vi "Uframe-QImg-MNR.vi"() -> ()   [LabVIEW 2010]
uses:
  <vilib>/Platform/TimedLoop/XDataNode/XDataNode.xnode
  <vilib>/Platform/TimedLoop/XDataNode/timing_clust.ctl
  <vilib>/Platform/TimedLoop/XDataNode/nitl_modes.ctl
  <vilib>/Platform/TimedLoop/XDataNode/wakeup.ctl
  <vilib>/Platform/TimedLoop/XDataNode/XDNodeRunTimeDep.lvlib
panel:
  out "Current Exposure":dbl
  out "Current Offset":dbl(slide)=1080.0 min=0.0 max=4095.0 step=1.0 scale=0.0..4095.0
  out "Current Gain":dbl(slide)=1100.0 min=0.0 max=4095.0 step=1.0 scale=0.0..4095.0
  in  "AE":bool
  in  "Offset":dbl(slide)=1080.0 min=0.0 max=4095.0 step=1.0 scale=0.0..4095.0
  out "All Stop":bool=TRUE
  out "QImage":T1(plugin-control)
  in  "Gain":dbl(slide)=1100.0 min=0.0 max=4095.0 step=1.0 scale=0.0..4095.0
  in  "Exposure (ms)":dbl(slide)=100.0 min=1.6 max=10000.0 step=0.001 scale=1.6..10000.0
  out "Load Cell Constant (N/V)":dbl=44.48
  in  "Load Cell":u16(ring)=1 items=["440 N", "1250 N"]
  in  "Pause @ Load":bool
  in  "Pause @ N":dbl
  out "Disp (mm)":dbl
  out "Load (N)":dbl
  out "Image #":i32
  in  "Illumination":u32(ring) items=["White Light", "Flourescent"]
  in  "Timed \nAcquisition":bool
  out "Data Point":i32
  in  "Data \nAcquisition \nInterval (s)":dbl=1.0 min=0.1 max=60.0
  in  "Capture\nCurrent Image":bool
  in  "Max Load (N)":dbl=600.0 min=0.0 max=1200.0
  out "At Limit":bool
  in  "Rate Multiplier":dbl=1.0
  in  "Pause \nDisplacement":bool
  in  "Stop":bool
  in  "Invert \nDisplacement":bool
  in  "Zero \nDisplacement":bool=TRUE
  in  "Begin":bool
  out "Load vs Disp":cluster{dbl[], dbl[]}(graph)={[-724.1250113144533, -724.195323815552, -724.2656363166506, -724.3359488177492, -724.4062613188479, -724.4765738199465, -724.5468863210451, -724.6171988221438, -724.7461050741579, -724.9218863269045, -725.0976675796511, -725.2851675825808, -725.4492300851442], [-11.89350874713131, -11.896152101474941, -11.894229661847117, -11.89350874707076, -11.890865392620372, -11.895671491596438, -11.895911796524977, -11.899756675680168, -11.899035760801853, -11.90552399441818, -11.907927043887174, -11.905283689458143, -11.914655582386047]}
  out "Disp Vs Time":cluster{dbl[], dbl[]}(graph)={[-724.1250113144533, -724.195323815552, -724.2656363166506, -724.3359488177492, -724.4062613188479, -724.4765738199465, -724.5468863210451, -724.6171988221438, -724.7461050741579, -724.9218863269045, -725.0976675796511, -725.2851675825808, -725.4492300851442], [-11.89350874713131, -11.896152101474941, -11.894229661847117, -11.89350874707076, -11.890865392620372, -11.895671491596438, -11.895911796524977, -11.899756675680168, -11.899035760801853, -11.90552399441818, -11.907927043887174, -11.905283689458143, -11.914655582386047]}
  in  "File Name":string="Test"
  in  "File Path":path=path "C:/cygwin/home/Smarter Materials/Users 2015/Michael Rossol"
  in  "Sample Notes":string
  in  "Displacement \nRate (um/s)":dbl=3.0 min=3.0 max=50.0
  in  "Data Acquisition \nInterval (s)":dbl=1.0 min=0.1 max=10.0 step=0.01 format="%#_3g"
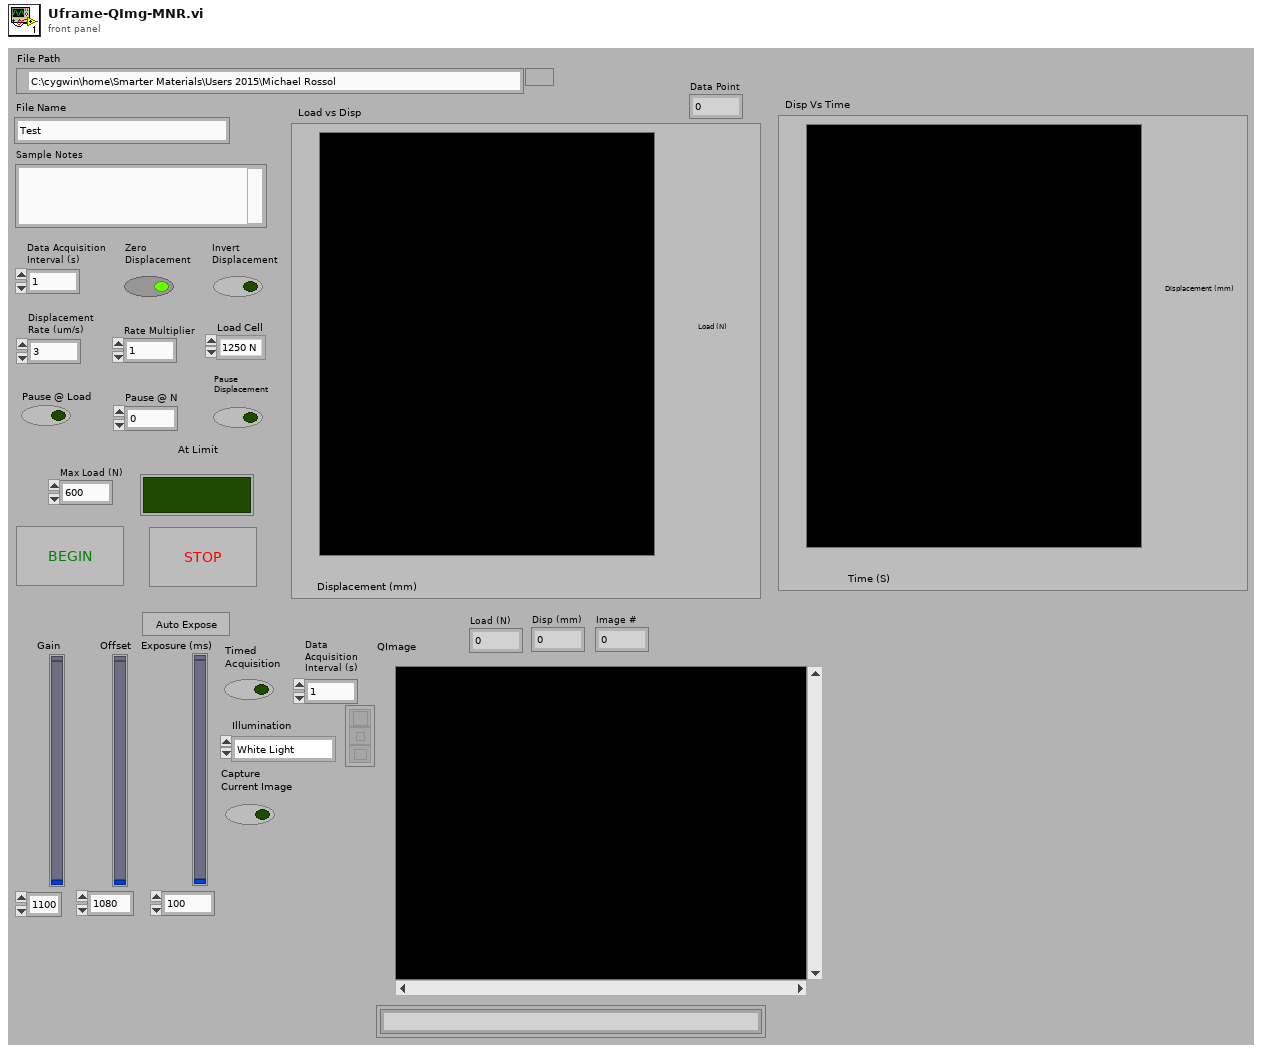
[diagram p1: front panel]
types:
  T1 = typedef "IMAQ Image.ctl" = refnum<image>
  T2 = enum32{"gain", "offset", "exposure", "binning", "horizontal binning", "vertical binning", "readout speed", "trigger type", "lcd filter", "cooler", "exposure red", "exposure blue", "image format", "roi x", "roi y", "roi width", "roi height", "reserved1", "shutter state", "reserved2", "sync-b out", "reserved3", "intensifier gain", "trigger delay", "camera mode", "normalized gain", "normalized intenifier gain DB", "doPostProcessing", "postProcessGainRed", "postProcessGainGreen", "postProcessGainBlue", "postProcessBayerAlgorithm", "postProcessImageFormat", "fan", "blackout mode", "high sensitivity", "Readout Port", "EM Gain", "open delay", "close delay", "clearing mode"}
  T3 = typedef "Image Type" = u32
  T4 = typedef "XDNodeRunTimeDep.lvlib/timing_clust.ctl" = cluster{"Expected End [f-1]":u64, "Actual End [f-1]":u64, "Finished Late? [f-1]":bool, "Expected End [i-1]":u64, "Actual End [i-1]":u64, "Finished Late? [i-1]":bool, "Expected Start [i]":u64, "Actual Start [i]":u64, "Expected Start [f]":u64, "Actual Start [f]":u64, "Source Name":string, "Structure Name":string, "Period":i64, "Deadline":i64, "Offset":i64, "Start":i64, "Priority":i32, "Timeout":i32, "Mode":T5, "Wakeup Reason":T6, "Error":errorcluster, "Source Type":string, "Secondary Source Type":string, "Global End Time":u64, "Global Start Time":u64, "Frame Duration":u64, "Iteration Duration":u64, "Assigned CPU":i32, "I/O Scan Engine Mode":u32}
  T5 = typedef "XDNodeRunTimeDep.lvlib/nitl_modes.ctl" = enum32{"No Change", "Process missed periods, maintain original phase", "Discard missed periods, maintain original phase", "Process missed periods, ignore original phase", "Discard missed periods, ignore original phase"}
  T6 = typedef "XDNodeRunTimeDep.lvlib/wakeup.ctl" = enum32{"Normal", "Aborted", "Asynchronous wakeup", "Timing source error", "Timed loop error", "Timeout"}
  T7 = cluster{"Global Rectangle":i32[], "Contours":cluster{"Contour Type":u32, "ROI Type":u32, "Points":i32[]}[]}
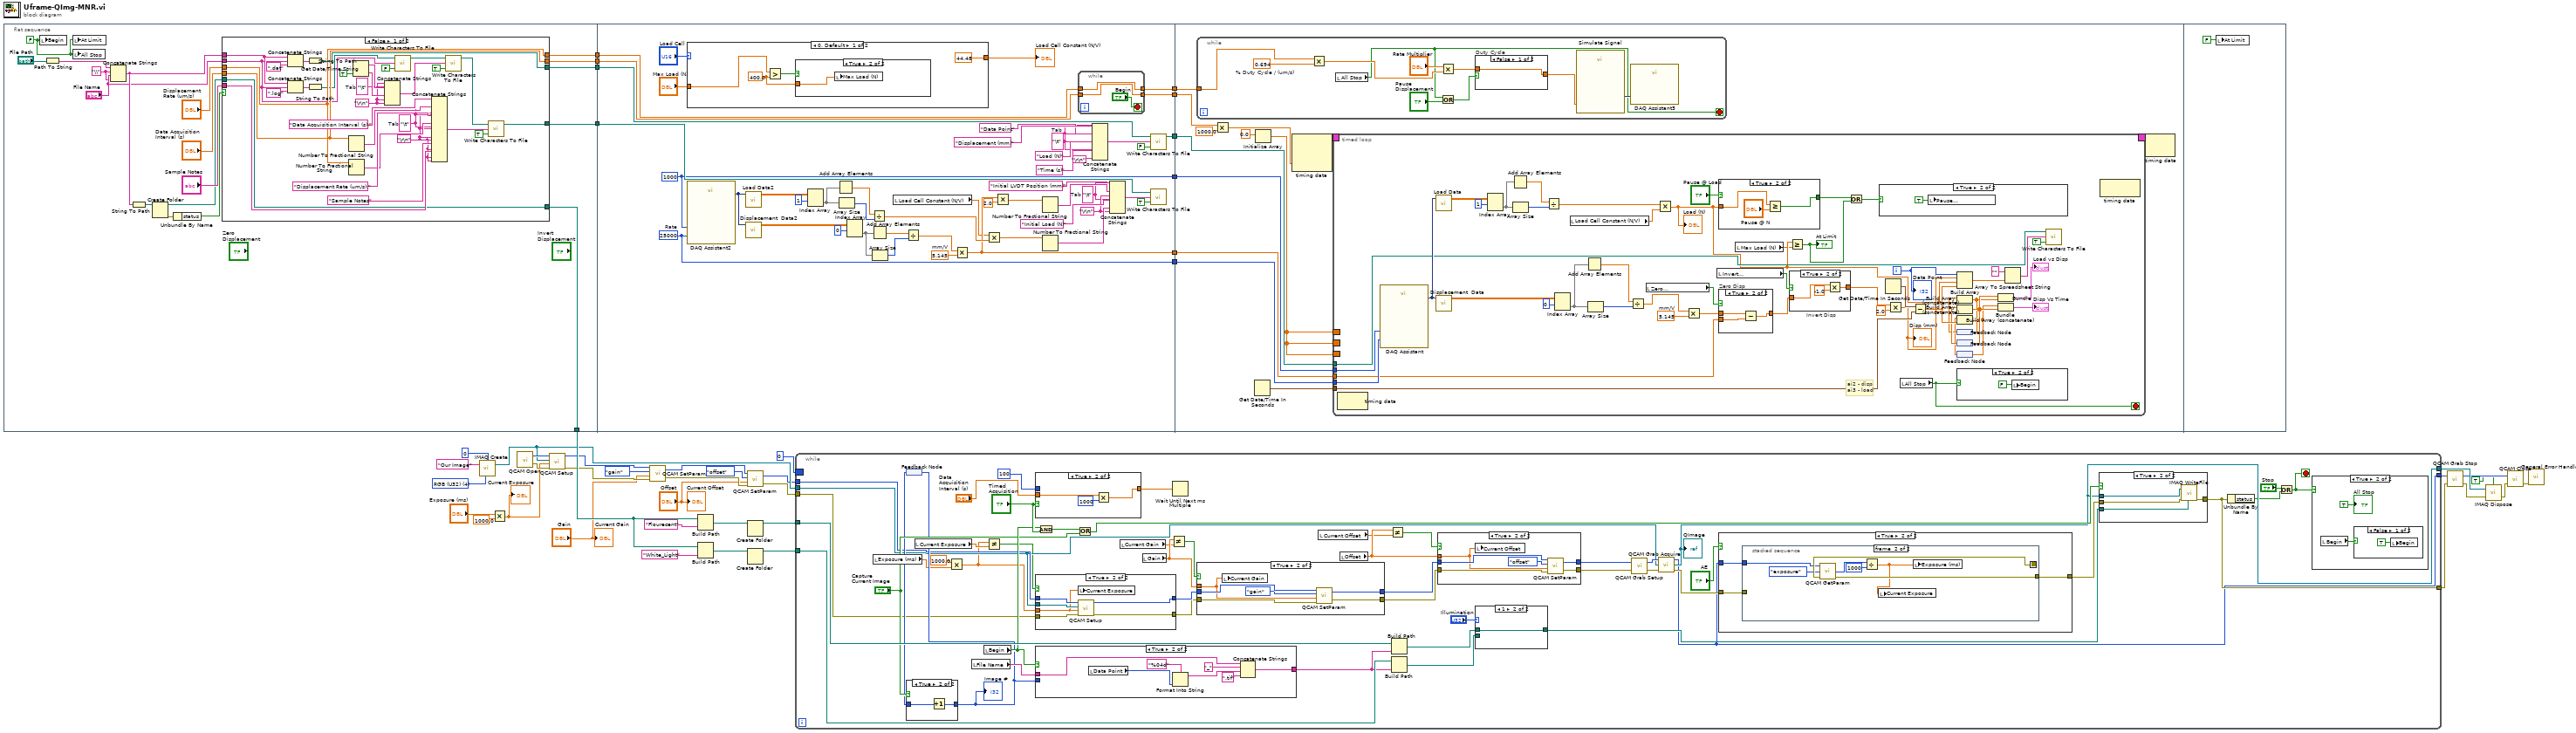
[diagram p0: block diagram]
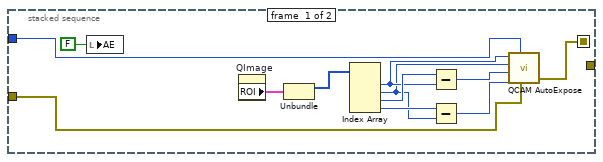
[diagram p6: hidden frame]
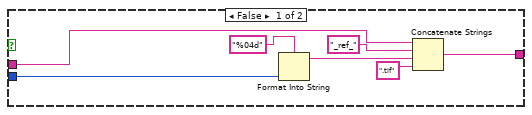
[diagram p10: hidden frame]
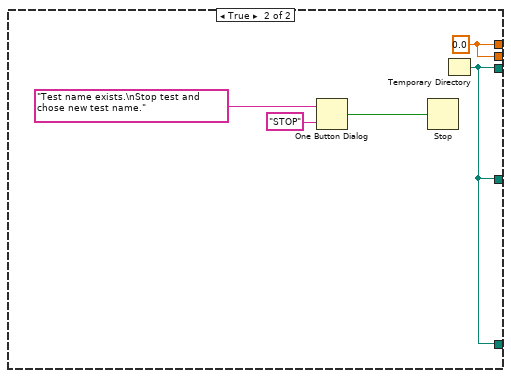
[diagram p14: hidden frame]
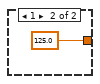
[diagram p16: hidden frame]
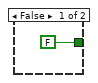
[diagram p17: hidden frame]
diagram:
  w21 = T3 4 items=["Grayscale (U8)", "Grayscale (I16)", "Grayscale (SGL)", "Complex (CSG)", "RGB (U32)", "HSL (U32)", "RGB (U64)"] ("Image Type")
  n1 = flat-sequence {
    tunnel: [w50] -> w41
    tunnel: [w62] -> w39
    tunnel: [w51] -> w38
    tunnel: [w52] -> w36
    tunnel: [w48] -> w29
    tunnel: [w105] -> w45
    tunnel: [w106] -> w44
    tunnel: [w107] -> w43
    tunnel: [w112] -> w42
    tunnel: w41 -> [w126]
    tunnel: [w117] -> w40
    tunnel: w39 -> [w116]
    tunnel: w38 -> [w109]
    tunnel: [w108] -> w37
    tunnel: w36 -> [w110]
    tunnel: w45 -> [w158]
    tunnel: w44 -> [w169]
    tunnel: w43 -> [w168]
    tunnel: w42 -> [w167]
    tunnel: w40 -> [w166]
    tunnel: w37 -> [w165]
    frame #0 {
      w49 = FALSE ("Begin")
      w47 = "\\"
      n2 = local write "Begin"(w49) -> ()
      n3 = Path To String(path="File Path") -> (string=w57:string)
      n4 = local write "At Limit"(w49) -> ()
      n5 = local write "All Stop"(w49) -> ()
      n6 = Concatenate Strings(w57, w47, "File Name", w47) -> (w55:string)
      n7 = String To Path(string=w55) -> (path=w59:path)
      n8 = Create Folder(path (use dialog)=w59) -> (created path=w46:path, error out=w58:errorcluster)  [unwired: 2 in, 1 out]
      n9 = Unbundle By Name(w58) -> ("status"=w56:bool)
      n10 = case shown="False" w56 {
        tunnel: [w81 w97] -> w50
        tunnel: "Data Acquisition \nInterval (s)" -> [w76 _]
        tunnel: "Displacement \nRate (um/s)" -> [w77 _]
        tunnel: "Sample Notes" -> [w73 _]
        tunnel: [w78 w97] -> w62
        tunnel: [w77 w96] -> w51
        tunnel: [w76 w96] -> w52
        tunnel: w55 -> [w66 _]
        tunnel: "File Name" -> [w65 _]
        tunnel: [w64 w97] -> w48
        tunnel: w46 -> [w64 _]
        frame False {
          w75 = "\t"  # Tab
          w72 = "\r\n"
          w91 = "\t"  # Tab
          w86 = "\r\n"
          n11 = Concatenate Strings(w66, w65, ".dat") -> (w79:string)
          n12 = Concatenate Strings(w66, w65, ".log") -> (w68:string)
          n13 = String To Path(string=w79) -> (path=w78:path)
          n14 = String To Path(string=w68) -> (path=w67:path)
          n15 = Number To Fractional String(number=w76) -> (F-format string=w84:string)  [unwired: 3 in]
          n16 = Number To Fractional String(number=w77) -> (F-format string=w82:string)  [unwired: 3 in]
          n17 = Get Date/Time String(want seconds? (F)=TRUE) -> (date string=w94:string, time string=w93:string)  [unwired: 2 in]
          n18 = Concatenate Strings(w86, w94, w91, w93, w86, w86) -> (w95:string)
          n19 = call <vilib>:"Write Characters To File.vi"("append to file? (new file:F)"=FALSE, "character string"=w65, "file path (dialog if empty)"=w67) -> ("new file path (Not A Path if cancelled)"=w71:path)  [unwired: 2 in]
          n20 = Concatenate Strings("Data Acquisition Interval (s):", w75, w84, w72, "Displacement Rate (um/s):", w75, w82, w72, w75, w72, w72, "Sample Notes", w72, w73, w72, w72) -> (w87:string)
          n21 = call <vilib>:"Write Characters To File.vi"("append to file? (new file:F)"=TRUE, "character string"=w95, "file path (dialog if empty)"=w71) -> ("new file path (Not A Path if cancelled)"=w89:path)  [unwired: 2 in]
          n22 = call <vilib>:"Write Characters To File.vi"("append to file? (new file:F)"=TRUE, "character string"=w87, "file path (dialog if empty)"=w89) -> ("new file path (Not A Path if cancelled)"=w81:path)  [unwired: 2 in]
        }
        frame True {
          w96 = 0.0 ("Displacement Rate (um/s)")
          n23 = One Button Dialog(message="Test name exists.\nStop test and chose new test name.", button name ("OK")="STOP") -> (true=w98:bool)
          n24 = Stop(stop? (T)=w98) -> ()
          n25 = Temporary Directory() -> (w97:path)
        }
      }
    }
    frame #1 {
      w107 = 1000 ("number of samples")
      w119 = "\t"  # Tab
      w130 = "\r\n"
      w128 = "\t"  # Tab
      w144 = 5.145  # mm/V
      w106 = 25000  # Rate
      n26 = case shown="0, Default" "Load Cell" {
        tunnel: [44.48 125.0] -> w103
        tunnel: "Max Load (N)" -> [w149 _]
        frame 0, Default {
          w148 = 400.0 ("y")
          n27 = Greater?(x=w149, y=w148) -> (0:w150:bool)
          n28 = case shown="True" w150 {
            tunnel: w148 -> [_ w152]
            frame False {
            }
            frame True {
              n29 = local write "Max Load (N)"(w152) -> ()
            }
          }
        }
        frame 1 {
        }
      }
      "Load Cell Constant (N/V)" <- w103
      n30 = call "DAQ Assistant2"("rate"=w106, "number of samples"=w107) -> ("data"=w135:dynamicdata)  [unwired: 15 in, 2 out]
      n31 = call "Load Data2"("Dynamic Data Type"=w135) -> ("Array"=w136:dbl[][])  [unwired: 3 in]
      n32 = call "Displacement  Data2"("Dynamic Data Type"=w135) -> ("Array"=w139:dbl[][])  [unwired: 3 in]
      n33 = Index Array(array=w136, index (row)=1) -> (element=w147:dbl[])  [unwired: 1 in]
      n34 = Add Array Elements(numeric array=w147) -> (sum=w145:dbl)
      n35 = Array Size(array=w147) -> (size(s)=w146:i32)
      n36 = Index Array(array=w139, index (row)=0) -> (element=w140:dbl[])  [unwired: 1 in]
      n37 = Divide(x=w145, y=w146) -> (x/y=w114:dbl)
      n38 = Add Array Elements(numeric array=w140) -> (sum=w141:dbl)
      n39 = Array Size(array=w140) -> (size(s)=w142:i32)
      n40 = local read "Load Cell Constant (N/V)"() -> (w104:dbl)
      n41 = Divide(x=w141, y=w142) -> (x/y=w143:dbl)
      n42 = Multiply(x=w143, y=w144) -> (x*y=w112:dbl)
      n43 = Multiply(x=w104, y=w114) -> (x*y=w115:dbl)
      n44 = Multiply(x=w112, y=2.0) -> (x*y=w113:dbl)
      n45 = Number To Fractional String(number=w113) -> (F-format string=w129:string)  [unwired: 3 in]
      n46 = Number To Fractional String(number=w115) -> (F-format string=w132:string)  [unwired: 3 in]
      n47 = while {
        tunnel: w109 -> [w155]
        tunnel: [w155] -> w108
        tunnel: [w154] -> w105
        tunnel: w110 -> [w154]
        stop <- "Begin" stop-if-true
      }
      n48 = Concatenate Strings("Data Point", w119, "Displacement (mm)" ("Substring"), w119, "Load (N)", w119, "Time (s)" ("string"), w119, "\r\n") -> (w124:string)
      n49 = Concatenate Strings("Initial LVDT Position (mm)", w128, w129, w130, "Initial Load (N)", w128, w132, w130) -> (w133:string)
      n50 = call <vilib>:"Write Characters To File.vi"("append to file? (new file:F)"=FALSE, "character string"=w124, "file path (dialog if empty)"=w116) -> ("new file path (Not A Path if cancelled)"=w117:path)  [unwired: 2 in]
      n51 = call <vilib>:"Write Characters To File.vi"("append to file? (new file:F)"=TRUE, "character string"=w133, "file path (dialog if empty)"=w126) -> ()  [unwired: 2 in, 1 out]
    }
    frame #2 {
      n52 = while {
        tunnel: w165 -> [w246]
        stop <- w239 stop-if-true
        w240 = 0.694  # % Duty Cycle / (um/s)
        n53 = Multiply(x=w246, y=w240) -> (x*y=w243:dbl)
        n54 = local read "All Stop"() -> (w239:bool)
        n55 = Multiply(x="Rate Multiplier", y=w243) -> (x*y=w242:dbl)
        n56 = Or(x=w239, y="Pause \nDisplacement") -> (x .or. y?=w245:bool)
        n57 = case "Duty Cycle" shown="False" w245 {
          tunnel: [w249 0.0 ("Duty Cycle (%)")] -> w247
          tunnel: w242 -> [w249 _]
          frame False {
          }
          frame True {
          }
        }
        n58 = call "Simulate Signal"("Duty Cycle (%)"=w247) -> ("Square"=w248:dynamicdata)  [unwired: 13 in, 1 out]
        n59 = call "DAQ Assistant3"("data"=w248) -> ()  [unwired: 16 in, 3 out]
      }
      n60 = Multiply(x=w158, y=1000.0) -> (x*y=w159:dbl)
      n61 = Get Date/Time In Seconds() -> (seconds since 1Jan1904=w162:timestamp)
      n62 = Initialize Array(0.0) -> (w163:dbl[])  [unwired: 1 in]
      n63 = node-c288(w159) -> (w161:T4)  [unwired: 2 in]
      n64 = timed-loop {
        tunnel: w168 -> [w201]
        tunnel: w169 -> [w200]
        tunnel: w167 -> [w192]
        tunnel: w162 -> [w196]
        tunnel: w166 -> [w195]
        border: w163 -> [_]
        border: w163 -> [_]
        border: w163 -> [_]
        timing: w161 -> [_]
        timing-out: [_] -> w160
        i -> [w178]
        stop <- w170 stop-if-true
        w199 = 5.145  # mm/V
        # "ai2 - disp\nai3 - load"
        n65 = node-c288() -> ()  [unwired: 1 in, 1 out]
        n66 = call "DAQ Assistant"("rate"=w200, "number of samples"=w201) -> ("data"=w198:dynamicdata)  [unwired: 15 in, 2 out]
        n67 = call "Load Data"("Dynamic Data Type"=w198) -> ("Array"=w213:dbl[][])  [unwired: 3 in]
        n68 = call "Displacement  Data"("Dynamic Data Type"=w198) -> ("Array"=w210:dbl[][])  [unwired: 3 in]
        n69 = Index Array(array=w213, index (row)=1) -> (element=w202:dbl[])  [unwired: 1 in]
        n70 = Add Array Elements(numeric array=w202) -> (sum=w204:dbl)
        n71 = Array Size(array=w202) -> (size(s)=w203:i32)
        n72 = Divide(x=w204, y=w203) -> (x/y=w189:dbl)
        n73 = Index Array(array=w210, index (row)=0) -> (element=w208:dbl[])  [unwired: 1 in]
        n74 = local read "Load Cell Constant (N/V)"() -> (w172:dbl)
        n75 = Add Array Elements(numeric array=w208) -> (sum=w207:dbl)
        n76 = Array Size(array=w208) -> (size(s)=w206:i32)
        n77 = Divide(x=w207, y=w206) -> (x/y=w205:dbl)
        n78 = local read "Zero \nDisplacement"() -> (w190:bool)
        n79 = Multiply(x=w189, y=w172) -> (x*y=w174:dbl)
        "Load (N)" <- w174
        n80 = Multiply(x=w205, y=w199) -> (x*y=w194:dbl)
        n81 = local read "Invert \nDisplacement"() -> (w191:bool)
        n82 = case shown="True" "Pause @ Load" {
          tunnel: w174 -> [_ w221]
          tunnel: [FALSE w220] -> w173
          frame False {
          }
          frame True {
            n83 = Greater Or Equal?(x=w221, y="Pause @ N") -> (x >= y?=w220:bool)
          }
        }
        n84 = case "Zero Disp" shown="True" w190 {
          tunnel: w192 -> [_ w234]
          tunnel: w194 -> [w231 w233]
          tunnel: [w231 w232] -> w193
          frame False {
          }
          frame True {
            n85 = Subtract(x=w233, y=w234) -> (x-y=w232:dbl)
          }
        }
        n86 = local read "Max Load (N)"() -> (w171:dbl)
        n87 = Greater Or Equal?(x=w174, y=w171) -> (x >= y?=w176:bool)
        "At Limit" <- w176
        n88 = case "Invert Disp" shown="True" w191 {
          tunnel: w193 -> [w227 w230]
          tunnel: [w227 w229] -> w187
          frame False {
          }
          frame True {
            n89 = Multiply(x=w230, y=-1.0) -> (x*y=w229:dbl)
          }
        }
        n90 = Or(x=w173, y=w176) -> (x .or. y?=w177:bool)
        n91 = case shown="True" w177 {
          frame False {
          }
          frame True {
            n92 = local write "Pause \nDisplacement"(TRUE ("Pause \nDisplacement")) -> ()
          }
        }
        n93 = Get Date/Time In Seconds() -> (seconds since 1Jan1904=w209:timestamp)
        n94 = Multiply(x=w187, y=2.0) -> (x*y=w186:dbl)
        "Disp (mm)" <- w186
        n95 = local read "All Stop"() -> (w170:bool)
        n96 = Subtract(x=w209, y=w196) -> (x-y=w197:dbl)
        n97 = Build Array(w178, w186, w174, w197) -> (w215:dbl[])
        n98 = feedback #1() -> (w181:dbl[])
        n99 = Build Array (concatenate)(w181, w174) -> (w182:dbl[])
        n100 = feedback-in #1(w182) -> ()
        n101 = feedback #2() -> (w183:dbl[])
        n102 = Build Array (concatenate)(w183, w186) -> (w184:dbl[])
        n103 = feedback-in #2(w184) -> ()
        n104 = feedback #3() -> (w179:dbl[])
        n105 = Build Array (concatenate)(w179, w197) -> (w180:dbl[])
        n106 = feedback-in #3(w180) -> ()
        n107 = case shown="True" w170 {
          frame False {
          }
          frame True {
            n108 = local write "Begin"(FALSE ("Begin")) -> ()
          }
        }
        n109 = Bundle(w184, w182) -> (→"Load vs Disp":cluster{dbl[], dbl[]})  [unwired: 1 in]
        n110 = Bundle(w180, w184) -> (→"Disp Vs Time":cluster{dbl[], dbl[]})  [unwired: 1 in]
        n111 = Array To Spreadsheet String(array=w215, 3:"" ("format string")) -> (spreadsheet string=w217:string)  [unwired: 1 in]
        n112 = call <vilib>:"Write Characters To File.vi"("append to file? (new file:F)"=TRUE, "character string"=w217, "file path (dialog if empty)"=w195) -> ()  [unwired: 2 in, 1 out]
        n113 = node-c288() -> ()  [unwired: 1 in, 1 out]
        "Data Point" <- w178
      }
      n114 = node-c288(w160) -> ()  [unwired: 1 out]
    }
    frame #3 {
      n115 = local write "At Limit"(FALSE ("Begin")) -> ()
    }
  }
  n116 = call "IMAQ Create"("Border Size"=0, "Image Name"="Our Image", "Image Type"=w21) -> ("New Image"=w11:T1)  [unwired: 2 in, 1 out]
  n117 = Multiply(x="Exposure (ms)", y=1000.0 ("x")) -> (x*y=w12:dbl)
  "Current Exposure" <- w12
  n118 = call <userlib>:"QCAM Open.vi"() -> ("error out"=w15:errorcluster, "cameraId out"=w16:u32)  [unwired: 2 in]
  n119 = call <userlib>:"QCAM Setup.vi"("error in (no error)"=w15, "Optional Exposure"=w12, "Image"=w11, "cameraId"=w16) -> ("error out"=w9:errorcluster, "cameraId out"=w10:u32)  [unwired: 3 in, 3 out]
  n120 = call <userlib>:"QCAM SetParam.vi"("error in (no error)"=w9, "value"="Gain", "parameter key"=T2."gain", "cameraId"=w10) -> ("error out"=w8:errorcluster, "cameraId out"=w7:u32)
  n121 = Build Path(base path=w29, name or relative path="Flourecent") -> (appended path=w30:path)
  n122 = Build Path(base path=w29, name or relative path="White_Light") -> (appended path=w33:path)
  n123 = call <userlib>:"QCAM SetParam.vi"("error in (no error)"=w8, "value"="Offset", "parameter key"=T2."offset", "cameraId"=w7) -> ("error out"=w5:errorcluster, "cameraId out"=w6:u32)
  n124 = Create Folder(path (use dialog)=w30) -> (created path=w28:path)  [unwired: 2 in, 2 out]
  n125 = Create Folder(path (use dialog)=w33) -> (created path=w32:path)  [unwired: 2 in, 2 out]
  n126 = while {
    tunnel: [w300] -> w20
    tunnel: [w281] -> w27
    tunnel: w32 -> [w294]
    tunnel: w28 -> [w292]
    border: 0 -> [_]
    tunnel: w11 -> [w266]
    tunnel: [w271] -> w23
    tunnel: w5 -> [w267]
    tunnel: w6 -> [w268]
    stop <- w278 stop-if-true
    n127 = local read "Exposure (ms)"() -> (w270:dbl)
    n128 = feedback #4() -> (w283:i32)
    n129 = case shown="True" "Capture\nCurrent Image" {
      tunnel: w283 -> [w351 w353]
      tunnel: [w351 w352] -> w282
      frame False {
      }
      frame True {
        n130 = Increment(x=w353) -> (x+1=w352:i32)
      }
    }
    "Image #" <- w282
    n131 = feedback-in #4(w282) -> ()
    n132 = local read "Current Exposure"() -> (w269:dbl)
    n133 = Multiply(x=1000.0, y=w270) -> (x*y=w264:dbl)
    n134 = local read "File Name"() -> (w285:string)
    n135 = local read "Begin"() -> (w287:bool)
    n136 = Not Equal?(x=w264, y=w269) -> (x != y?=w265:bool)
    n137 = case shown="True" "Timed \nAcquisition" {
      tunnel: u32 100 ("y") -> [w370 _]
      tunnel: [w370 w373] -> w298
      tunnel: "Data \nAcquisition \nInterval (s)" -> [_ w372]
      frame False {
      }
      frame True {
        n138 = Multiply(x=w372, y=1000) -> (x*y=w373:dbl)
      }
    }
    n139 = case shown="True" w265 {
      tunnel: w268 -> [w318 w324]
      tunnel: w267 -> [w317 w323]
      tunnel: w266 -> [_ w322]
      tunnel: [w318 w321] -> w263
      tunnel: [w317 w320] -> w262
      tunnel: w264 -> [_ w319]
      frame False {
      }
      frame True {
        n140 = local write "Current Exposure"(w319) -> ()
        n141 = call <userlib>:"QCAM Setup.vi"("error in (no error)"=w323, "Optional Exposure"=w319, "Image"=w322, "cameraId"=w324) -> ("error out"=w320:errorcluster, "cameraId out"=w321:u32)  [unwired: 3 in, 3 out]
      }
    }
    n142 = case shown="True" w287 {
      tunnel: [w358 w367] -> w286
      tunnel: w285 -> [w360 w366]
      tunnel: w282 -> [w356 _]
      frame False {
        n143 = Format Into String(format string="%04d", w356) -> (resulting string=w357:string)  [unwired: 2 in, 1 out]
        n144 = Concatenate Strings(w360, "_ref_" ("string"), w357, ".tif") -> (w358:string)
      }
      frame True {
        n145 = local read "Data Point"() -> (w361:i32)
        n146 = Format Into String(format string="%04d", w361) -> (resulting string=w363:string)  [unwired: 2 in, 1 out]
        n147 = Concatenate Strings(w366, "_" ("string"), w363, ".tif") -> (w367:string)
      }
    }
    n148 = And(x=w287, y="Timed \nAcquisition") -> (x .and. y?=w295:bool)
    n149 = Or(x=w295, y="Capture\nCurrent Image") -> (x .or. y?=w296:bool)
    n150 = local read "Current Gain"() -> (w259:dbl)
    n151 = local read "Gain"() -> (w261:dbl)
    n152 = Not Equal?(x=w261, y=w259) -> (x != y?=w260:bool)
    n153 = Wait Until Next ms Multiple(millisecond multiple=w298) -> ()  [unwired: 1 out]
    n154 = case shown="True" w260 {
      tunnel: w263 -> [w309 w316]
      tunnel: w262 -> [w310 w315]
      tunnel: [w310 w314] -> w255
      tunnel: [w309 w313] -> w258
      tunnel: w261 -> [_ w311]
      frame False {
      }
      frame True {
        n155 = local write "Current Gain"(w311) -> ()
        n156 = call <userlib>:"QCAM SetParam.vi"("error in (no error)"=w315, "value"=w311, "parameter key"=T2."gain", "cameraId"=w316) -> ("error out"=w314:errorcluster, "cameraId out"=w313:u32)
      }
    }
    n157 = local read "Current Offset"() -> (w253:dbl)
    n158 = local read "Offset"() -> (w254:dbl)
    n159 = Not Equal?(x=w254, y=w253) -> (x != y?=w252:bool)
    n160 = Build Path(base path=w292, name or relative path=w286) -> (appended path=w289:path)
    n161 = Build Path(base path=w294, name or relative path=w286) -> (appended path=w291:path)
    n162 = case shown="True" w252 {
      tunnel: w258 -> [w302 w308]
      tunnel: [w302 w307] -> w257
      tunnel: [w301 w306] -> w256
      tunnel: w255 -> [w301 w305]
      tunnel: w254 -> [_ w303]
      frame False {
      }
      frame True {
        n163 = local write "Current Offset"(w303) -> ()
        n164 = call <userlib>:"QCAM SetParam.vi"("error in (no error)"=w305, "value"=w303, "parameter key"=T2."offset", "cameraId"=w308) -> ("error out"=w306:errorcluster, "cameraId out"=w307:u32)
      }
    }
    n165 = case shown="1" "Illumination" {
      tunnel: w291 -> [w368 _]
      tunnel: [w368 w369] -> w290
      tunnel: w289 -> [_ w369]
      frame 0, Default {
      }
      frame 1 {
      }
    }
    n166 = call <userlib>:"QCAM Grab Setup.vi"("error in (no error)"=w256, "cameraId"=w257) -> ("error out"=w276:errorcluster, "cameraId out"=w277:u32)
    n167 = call <userlib>:"QCAM Grab Acquire.vi"("error in (no error)"=w276, "Image"=w266, "cameraId"=w277) -> ("error out"=w273:errorcluster, "Image Out"=w281:T1, "cameraId out"=w271:u32)
    "QImage" <- w281
    n168 = case shown="True" "AE" {
      tunnel: w273 -> [w325 w327]
      tunnel: w271 -> [_ w328]
      tunnel: [w325 w326] -> w272
      frame False {
      }
      frame True {
        n169 = stacked-sequence {
          seq-local: [w330 _] -> [_ w345]
          tunnel: w328 -> [w339 w343]
          tunnel: w327 -> [w331 _]
          tunnel: [_ w344] -> w326
          frame #0 {
            n170 = local write "AE"(FALSE) -> ()
            n171 = property on="QImage" class="ImageControl"() -> ("ROI"=w329:T7)  [unwired: 2 in, 2 out]
            n172 = Unbundle(w329) -> ("Global Rectangle"=w336:i32[])  [unwired: 1 out]
            n173 = Index Array(array=w336) -> (element #1=w333:i32, element #2=w332:i32, element #3=w335:i32, element #4=w334:i32)  [unwired: 4 in]
            n174 = Subtract(x=w335, y=w333) -> (x-y=w337:i32)
            n175 = Subtract(x=w334, y=w332) -> (x-y=w338:i32)
            n176 = call <userlib>:"QCAM AutoExpose.vi"("xOrig"=w333, "cameraId"=w339, "yOrig"=w332, "width"=w337, "error in (no error)"=w331, "height"=w338) -> ("error out"=w330:errorcluster)  [unwired: 1 in, 1 out]
          }
          frame #1 {
            n177 = call <userlib>:"QCAM GetParam.vi"("cameraId in"=w343, "parameter key"=T2."exposure", "error in (no error)"=w345) -> ("value out"=w347:u32, "error out"=w344:errorcluster)  [unwired: 3 out]
            n178 = Divide(x=w347, y=1000) -> (x/y=w341:dbl)
            n179 = local write "Current Exposure"(w341) -> ()
            n180 = local write "Exposure (ms)"(w341) -> ()
          }
        }
      }
    }
    n181 = case shown="True" w296 {
      tunnel: w281 -> [_ w378]
      tunnel: [w374 w377] -> w300
      tunnel: w290 -> [_ w376]
      tunnel: w272 -> [w374 w375]
      frame False {
      }
      frame True {
        n182 = call "IMAQ WriteFile"("error in (no error)"=w375, "File Path"=w376, "Image"=w378) -> ("error out"=w377:errorcluster)  [unwired: 5 in]
      }
    }
    n183 = Unbundle By Name(w300) -> ("status"=w280:bool)
    n184 = Or(x="Stop", y=w280) -> (x .or. y?=w278:bool)
    n185 = case shown="True" w278 {
      frame False {
      }
      frame True {
        n186 = local read "Begin"() -> (w348:bool)
        n187 = case shown="False" w348 {
          frame False {
            n188 = local write "Begin"(TRUE) -> ()
          }
          frame True {
          }
        }
        "All Stop" <- TRUE
      }
    }
  }
  n189 = call <userlib>:"QCAM Grab Stop.vi"("error in (no error)"=w20, "cameraId"=w23) -> ("error out"=w18:errorcluster, "cameraId Out"=w25:u32)
  n190 = call "IMAQ Dispose"("All Images? (No)"=TRUE, "Image"=w27, "error in (no error)"=w18) -> ("error out"=w17:errorcluster)  [unwired: 3 in]
  n191 = call <userlib>:"QCAM Close.vi"("error in (no error)"=w17, "cameraId"=w25) -> ("error out"=w26:errorcluster)  [unwired: 1 in]
  n192 = call <vilib>:"General Error Handler.vi"("error in (no error)"=w26) -> ()  [unwired: 10 in, 5 out]
  "Current Gain" <- "Gain"
  "Current Offset" <- "Offset"
